vi "Set_Array_Size.vi"(10 "ArraySizes":i32, 11 "ChillerNew.lvclass":refnum<class "ChillerNew.lvclass">) -> (3 "output cluster":refnum<class "ChillerNew.lvclass">)   [LabVIEW 2023]
uses:
  ChillerNew.lvclass
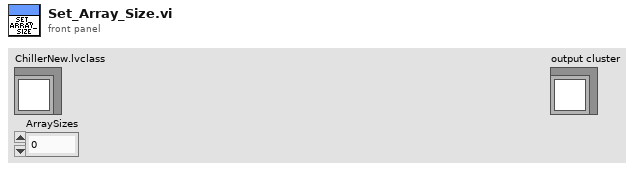
[diagram p1: front panel]
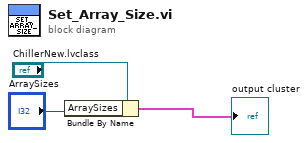
[diagram p0: block diagram]
diagram:
  n1 = Bundle By Name(cluster="ChillerNew.lvclass", "ArraySizes"="ArraySizes") -> (→"output cluster":cluster{})
